vi "Build Pass Message.vi"(10 "Test Name":string, 11 "Result":refnum<class "Abs_Double Float.lvclass">) -> (3 "Abs_String out":refnum<class "Abs_String.lvclass">)   [LabVIEW 2021, in "Test Sequencer Support.lvlib"]
uses:
  <vilib>/TSA/Abstract Data Classes/Abs_Types/Double Float/Abs_Double Float.lvclass
  C:/Program Files (x86)/National Instruments/LabVIEW 2021/vi.lib/TSA/Abstract Data Classes/Abs_Types/Value/Abs_Value.lvclass
  <vilib>/TSA/Abstract Data Classes/Abs_Types/String/Abs_String.lvclass
  <vilib>/TSA/Abstract Data Classes/Constants/Support/Str/Str.vi
  Test Sequencer Support.lvlib
  <vilib>/TSA/Abstract Data Classes/Constants/Support/Str/Const_Str.lvclass
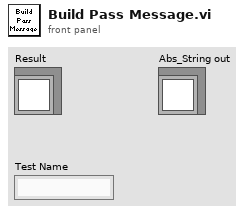
[diagram p1: front panel]
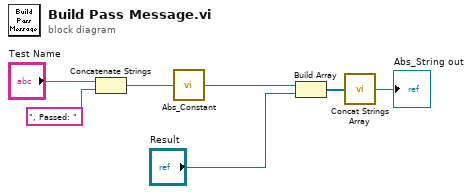
[diagram p0: block diagram]
diagram:
  n1 = Concatenate Strings("Test Name", ", Passed: " ("string")) -> (w2:string)
  n2 = call-poly <vilib>:"Abs_Constant.vi"("String"=w2) -> ("Abs_String.lvclass"=w6:refnum<class "Abs_String.lvclass">)  [unwired: 4 in]
  n3 = Build Array(w6, "Result") -> (w4:refnum<class "Abs_Value.lvclass">[])
  n4 = call <vilib>:"Concat Strings Array.vi"("Strings"=w4) -> ("Result"=→"Abs_String out":refnum<class "Abs_String.lvclass">)  [unwired: 4 in]
